vi "MainBancoEiettori.vi"() -> ()   [LabVIEW 2025]
uses:
  <vilib>/Utility/file.llb/Write Delimited Spreadsheet (DBL).vi
panel:
  out "_NewTest":bool
  out "Numeric":i32
  out "_InsertCase":bool
  out "Exit":bool
  in  "stop":bool
  out "array":dbl[][](array[numeric]) format="%#_5g"
  out "Outlet  [mA]":dbl
  out "Secondary [mA]":dbl
  out "Primary [mA]":dbl
  out "Outlet [bar]":dbl
  out "Secondary [bar]":dbl
  out "Primary [bar]":dbl
  in  "Insert Case":bool
  in  "New test":bool
  out "Waveform Chart":T1(graph)
  # "Actual Pressure Values"
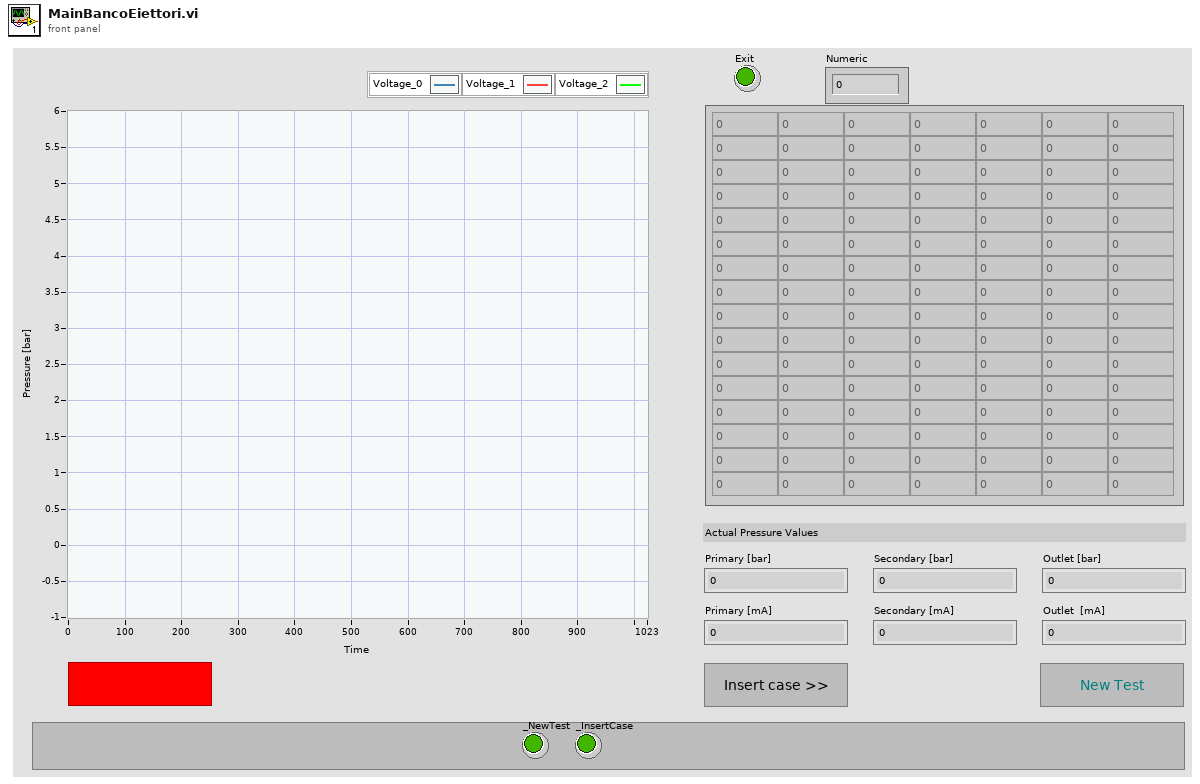
[diagram p1: front panel]
types:
  T1 = cluster{"Scalar":dbl, "Scalar":dbl, "Scalar":dbl}
  T2 = cluster{"Scalar":dbl, "Scalar":dbl, "Scalar":dbl}[]
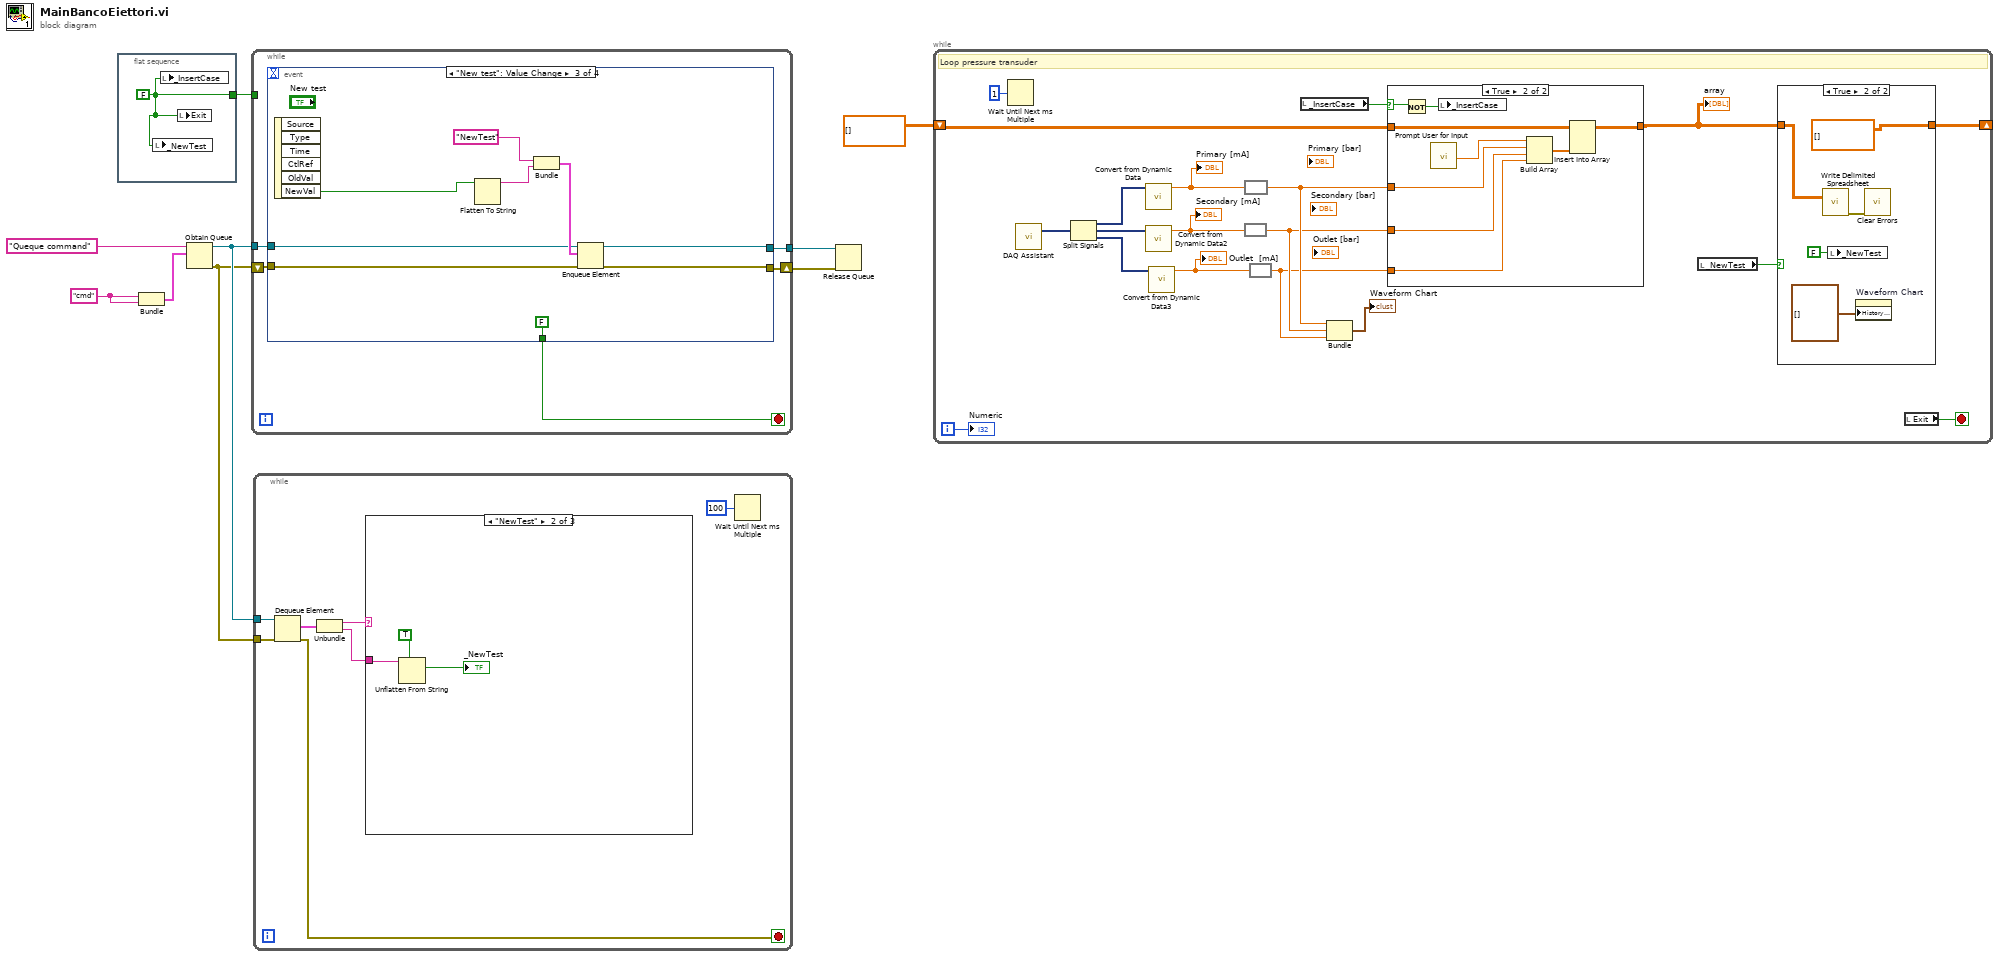
[diagram p0: block diagram]
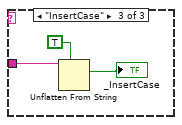
[diagram p5: hidden frame]
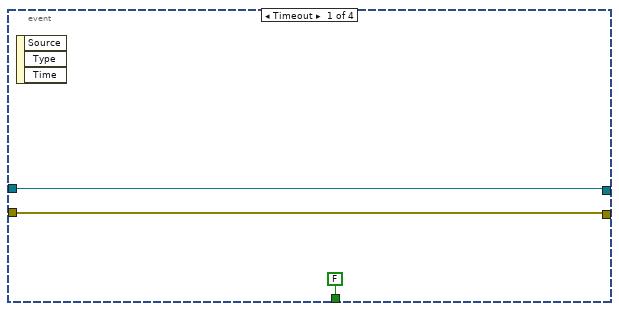
[diagram p6: hidden frame]
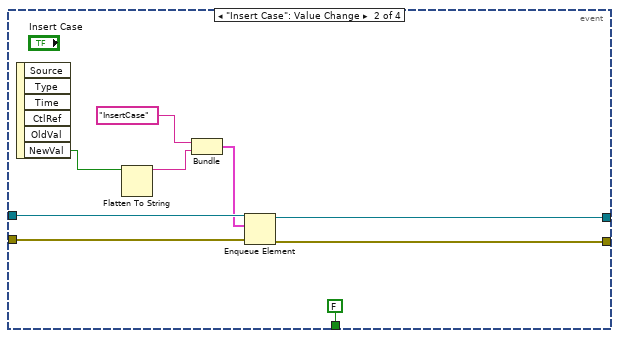
[diagram p7: hidden frame]
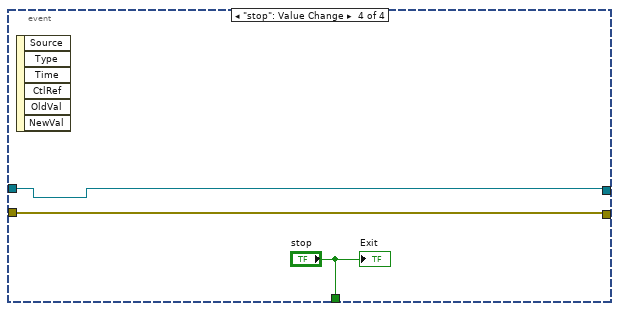
[diagram p8: hidden frame]
diagram:
  w2 = "cmd"
  n1 = flat-sequence {
    tunnel: [w10] -> w1
    frame #0 {
      w10 = FALSE ("_InsertCase 2")
      n2 = local write "_NewTest"(w10) -> ()
      n3 = local write "_InsertCase"(w10) -> ()
      n4 = local write "Exit"(w10) -> ()
    }
  }
  n5 = Bundle(w2, w2) -> (w7:cluster{string, string})  [unwired: 1 in]
  n6 = Obtain Queue(name (unnamed)="Queque command", element data type=w7) -> (queue out=w4:refnum<queue>, error out=w3:errorcluster)  [unwired: 3 in, 1 out]
  n7 = while {
    tunnel: w4 -> [w15]
    shift-right: [w13] -> w5
    shift-left: w3 -> [w14]
    tunnel: [w12] -> w6
    tunnel: w1 -> [_]
    stop <- w11 stop-if-true
    n8 = event shown="[2] \"New test\": Value Change" {
      selector: _ -> [_ _ _ _]
      dyn-events: _ -> [_ _ _ _]
      timeout: _ -> [_ _ _ _]
      tunnel: w15 -> [w18 w27 w32 w39]
      tunnel: w14 -> [w17 w26 w31 w38]
      tunnel: [w17 w25 w29 w38] -> w13
      tunnel: [w18 w24 w30 w39] -> w12
      tunnel: [FALSE ("stop") FALSE ("stop") FALSE ("stop") "stop"] -> w11
      event Timeout {
        n9 = event-data() -> ()  [unwired: 1 in, 3 out]
      }
      event "Insert Case": Value Change {
        n10 = event-data() -> ("NewVal"=w19:bool)  [unwired: 1 in, 5 out]
        n11 = Flatten To String(anything=w19) -> (data string=w22:string)  [unwired: 3 in, 2 out]
        n12 = Bundle("InsertCase", "data string"=w22) -> (w21:cluster{string, "data string":string})  [unwired: 1 in]
        n13 = Enqueue Element(queue=w27, element=w21, error in (no error)=w26) -> (queue out=w24:refnum<queue>, error out=w25:errorcluster)  [unwired: 1 in, 1 out]
      }
      event "New test": Value Change {
        n14 = event-data() -> ("NewVal"=w28:bool)  [unwired: 1 in, 5 out]
        n15 = Flatten To String(anything=w28) -> (data string=w34:string)  [unwired: 3 in, 2 out]
        n16 = Bundle("NewTest", "data string"=w34) -> (w33:cluster{string, "data string":string})  [unwired: 1 in]
        n17 = Enqueue Element(queue=w32, element=w33, error in (no error)=w31) -> (queue out=w30:refnum<queue>, error out=w29:errorcluster)  [unwired: 1 in, 1 out]
      }
      event "stop": Value Change {
        n18 = event-data() -> ()  [unwired: 1 in, 6 out]
        "Exit" <- "stop"
      }
    }
  }
  n19 = while {
    tunnel: w4 -> [w45]
    tunnel: w3 -> [w44]
    stop <- w40 stop-if-true
    n20 = Dequeue Element(queue=w45, error in (no error)=w44) -> (element=w43:cluster{string, string}, error out=w40:errorcluster)  [unwired: 1 in, 2 out]
    n21 = Unbundle(w43) -> (w42:string, w41:string)
    n22 = case shown="\"NewTest\"" w42 {
      tunnel: w41 -> [_ w48 w52]
      frame "False", Default {
      }
      frame "NewTest" {
        n23 = Unflatten From String(type=TRUE, binary string=w48) -> (value=→"_NewTest":bool)  [unwired: 3 in, 2 out]
      }
      frame "InsertCase" {
        n24 = Unflatten From String(type=TRUE, binary string=w52) -> (value=→"_InsertCase":bool)  [unwired: 3 in, 2 out]
      }
    }
    n25 = Wait Until Next ms Multiple(millisecond multiple=u32 100) -> ()  [unwired: 1 out]
  }
  n26 = Release Queue(queue=w6, error in (no error)=w5) -> ()  [unwired: 1 in, 3 out]
  n27 = while {
    shift-right: [w53] -> _
    shift-left: dbl[][] [] ("array") -> [w66]
    i -> [w60]
    stop <- w71 stop-if-true
    # "Loop pressure transuder"
    n28 = Wait Until Next ms Multiple(millisecond multiple=u32 1) -> ()  [unwired: 1 out]
    n29 = call "DAQ Assistant"() -> ("data"=w61:dynamicdata)  [unwired: 17 in, 2 out]
    n30 = Split Signals(w61) -> (w69:dynamicdata, w68:dynamicdata, w67:dynamicdata)  [unwired: 3 in]
    n31 = call "Convert from Dynamic Data"("Dynamic Data Type"=w69) -> ("Scalar"=w65:dbl)  [unwired: 3 in]
    "Primary [mA]" <- w65
    n32 = call "Convert from Dynamic Data2"("Dynamic Data Type"=w68) -> ("Scalar"=w64:dbl)  [unwired: 3 in]
    "Secondary [mA]" <- w64
    n33 = call "Convert from Dynamic Data3"("Dynamic Data Type"=w67) -> ("Scalar"=w63:dbl)  [unwired: 3 in]
    "Outlet  [mA]" <- w63
    n34 = expression code=""(w64) -> (w58:dbl)
    n35 = expression code=""(w65) -> (w59:dbl)
    n36 = expression code=""(w63) -> (w57:dbl)
    n37 = local read "_InsertCase"() -> (w62:bool)
    n38 = Bundle("Scalar"=w59, "Scalar"=w58, "Scalar"=w57) -> (→"Waveform Chart":T1)  [unwired: 1 in]
    n39 = case shown="True" w62 {
      selector: w62 -> [_ w80]
      tunnel: w59 -> [_ w86]
      tunnel: w58 -> [_ w85]
      tunnel: w57 -> [_ w84]
      tunnel: [w78 w87] -> w54
      tunnel: w66 -> [w78 w81]
      frame False {
      }
      frame True {
        n40 = Not(x=w80) -> (.not. x?=w79:bool)
        n41 = call "Prompt User for Input"() -> ("Current"=w82:dbl)  [unwired: 17 in, 2 out]
        n42 = local write "_InsertCase"(w79) -> ()
        n43 = Build Array(w82, w86, w85, w84) -> (w83:dbl[])
        n44 = Insert Into Array(array=w81, new element=w83) -> (w87:dbl[][])  [unwired: 2 in]
      }
    }
    "array" <- w54
    n45 = local read "_NewTest"() -> (w55:bool)
    n46 = case shown="True" w55 {
      tunnel: w54 -> [w72 w75]
      tunnel: [w72 dbl[][] [] ("array")] -> w53
      frame False {
      }
      frame True {
        n47 = call-poly <vilib>:"Write Delimited Spreadsheet.vi"("2D data"=w75) -> ("error out"=w73:errorcluster)  [unwired: 13 in, 1 out]
        n48 = local write "_NewTest"(FALSE ("_NewTest")) -> ()
        n49 = property on="Waveform Chart" class="WFChart (strict)"("History Data"=T2 []) -> ()  [unwired: 2 in, 2 out]
        n50 = call <vilib>:"Clear Errors.vi"("error in (no error)"=w73) -> ()  [unwired: 5 in, 2 out]
      }
    }
    n51 = local read "Exit"() -> (w71:bool)
    "Numeric" <- w60
  }
